vi "CODMn启动 (子VI).vi"(11 "启动测量模式":T2) -> (0 "error out":T1={"status"=FALSE, "代码"=4, "source"=""} caption="错误输出" {"代码" items=["执行成功"=1, "执行失败，但不知道原因"=2, "命令请求条件错误"=3, "通讯超时"=4, "系统繁忙不能执行"=5, "系统故障"=6, "没有数据"=100]})   [LabVIEW 2016]
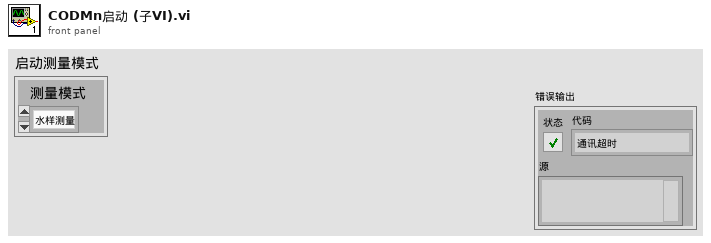
[diagram p1: front panel]
types:
  T1 = cluster{"status":bool, "代码":u16, "source":string}
  T2 = cluster{"测量模式":enum16{"水样测量", "标样核查", "零点核查", "跨度核查", "空白测试", "加标回收", "平行样", "校零", "校标"}}
  T3 = enum16{"空闲", "水样测试", "标样核查", "零点核查", "跨度核查", "空白测试", "平行样测试", "质控样", "空白校准", "标样校准", "加标回收"}
  T4 = cluster{"COD浓度（mg/L)":dbl, "水样启动时间":timestamp, "加标回收启动时间":timestamp, "CODMn工作状态":enum16{"空闲", "水样测试", "标样核查", "零点核查", "跨度核查", "空白测试", "平行样测试", "加标回收", "空白校准", "标样校准", "初始化（清洗）"}, "多列列表框":i32}
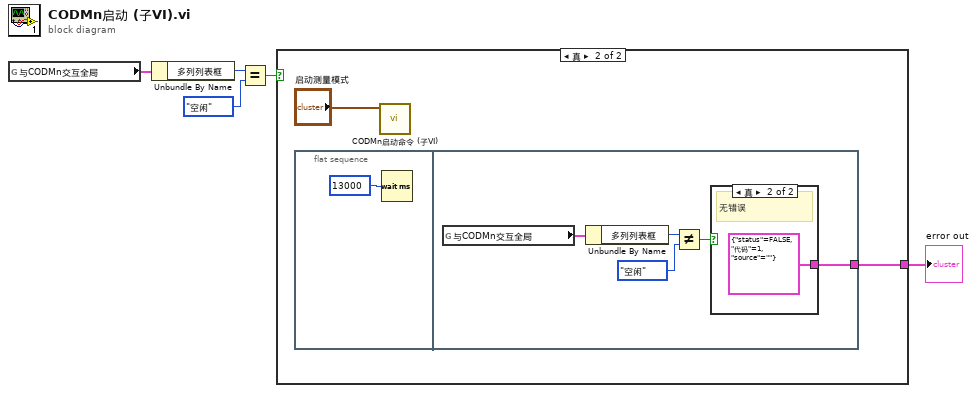
[diagram p0: block diagram]
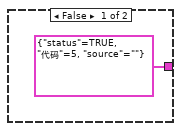
[diagram p2: hidden frame]
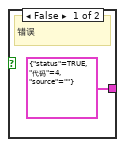
[diagram p3: hidden frame]
diagram:
  n1 = global read "modbus slave全局.vi" "与CODMn交互全局"() -> (w2:T4)
  n2 = Unbundle By Name(w2) -> ("多列列表框"=w1:i32)
  n3 = Equal?(x=w1, y=T3."空闲") -> (x = y?=w4:bool)
  n4 = case shown="真" w4 {
    tunnel: [T1 {"status"=TRUE, "代码"=5, "source"=""} ("error out") w8] -> w3
    frame False {
    }
    frame True {
      n5 = flat-sequence {
        tunnel: [w12] -> w8
        frame #0 {
          n6 = Wait (ms)(milliseconds to wait=u32 13000 ("等待时间（毫秒）")) -> ()  [unwired: 1 out]
        }
        frame #1 {
          n7 = global read "modbus slave全局.vi" "与CODMn交互全局"() -> (w11:T4)
          n8 = Unbundle By Name(w11) -> ("多列列表框"=w10:i32)
          n9 = Not Equal?(x=w10, y=T3."空闲") -> (x != y?=w13:bool)
          n10 = case shown="真" w13 {
            tunnel: [T1 {"status"=TRUE, "代码"=4, "source"=""} ("error out") T1 {"status"=FALSE, "代码"=1, "source"=""} ("error out")] -> w12
            frame False {
              # "错误"
            }
            frame True {
              # "无错误"
            }
          }
        }
      }
      n11 = call "CODMn启动命令 (子VI).vi"("启动测量模式"="启动测量模式") -> ()  [unwired: 11 in]
    }
  }
  "error out" <- w3
